vi "SetValue.vi"(8 "error in":errorcluster, 10 "Value":i64, 11 "IntergerMeasure in":refnum<class "IntegerMeasure.lvclass">) -> (0 "error out":errorcluster, 3 "IntergerMeasure out":refnum<class "IntegerMeasure.lvclass">)   [LabVIEW 2021, in "ProligentXMLGenerator.lvlib" / "IntegerMeasure.lvclass"]
doc: "Defines the value acquired by the measure."
uses:
  IntegerMeasure.lvclass
  IntegerMeasure.lvclass/IntegerMeasure.ctl
  Base/String_4000/String_4000.lvclass
  Base/Integer/Integer.lvclass
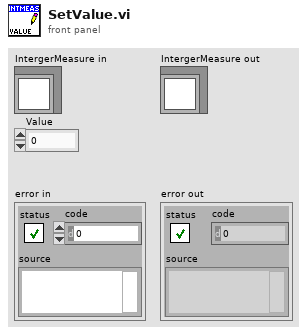
[diagram p1: front panel]
types:
  T1 = typedef "ProligentXMLGenerator.lvlib/IntegerMeasure.lvclass/Data.ctl" = cluster{"Value":refnum<class "Integer.lvclass">}
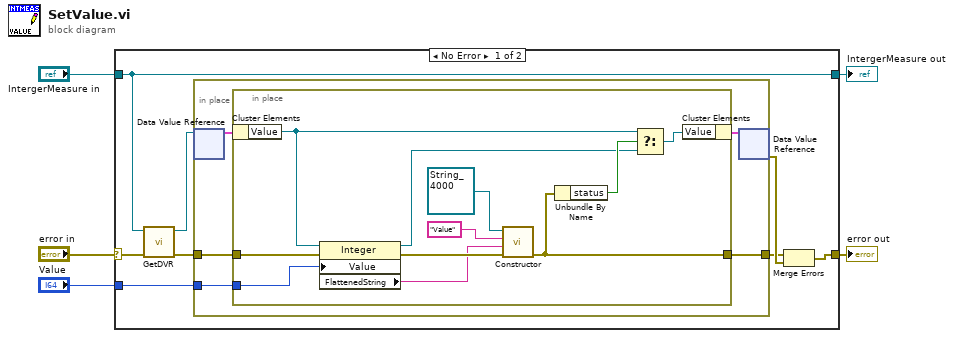
[diagram p0: block diagram]
diagram:
  n1 = case shown="No Error" "error in" {
    selector: "error in" -> [w6 w30]
    tunnel: "IntergerMeasure in" -> [w7 w31]
    tunnel: [w12 w30] -> w3
    tunnel: "Value" -> [w11 _]
    tunnel: [w7 w31] -> w1
    frame No Error {
      n2 = call "GetDVR.vi"("error in"=w6, "IntergerMeasure"=w7) -> ("error out"=w10:errorcluster, "DVRReference"=w13:refnum<data-value>)  [unwired: 8 in]
      n3 = in-place "In Place Element Structure" {
        in-place-border: w11 -> [w18]
        in-place-border: w10 -> [w15]
        in-place-border: [w14] -> w8
        n4 = in-place-dvr #1(w13) -> (w17:T1)  [unwired: 1 out]
        n5 = in-place "In Place Element Structure" {
          in-place-border: w18 -> [w21]
          in-place-border: w15 -> [w29]
          in-place-border: [w25] -> w14
          n6 = in-place-cluster #2(w17) -> ("Value"=w22:refnum<class "Integer.lvclass">)
          n7 = property on="Property Node" class="Integer"(reference=w22, error in=w29, "Value"=w21) -> (reference out=w19:refnum<class "Integer.lvclass">, error out=w27:errorcluster, "FlattenedString"=w20:string)
          n8 = call-dynamic "Constructor.vi"("error in"=w27, "Value"=w20, "Name"="Value", "String in"=refnum<class "String_4000.lvclass"> refnum ("ProligentResultProcessor:String_4000")) -> ("error out"=w25:errorcluster)  [unwired: 6 in, 1 out]
          n9 = Unbundle By Name(w25) -> ("status"=w24:bool)
          n10 = Select(t=w22, s=w24, f=w19) -> (s? t:f=w23:refnum<class "Integer.lvclass">)
          n11 = in-place-cluster #2("Value"=w23) -> (w16:T1)
        }
        n12 = in-place-dvr #1(w16) -> (w9:errorcluster)  [unwired: 1 out]
      }
      n13 = Merge Errors(w8, w9) -> (w12:errorcluster)
    }
    frame Error {
    }
  }
  "error out" <- w3
  "IntergerMeasure out" <- w1
